vi "variantCtrlIoType.vi"(4 "isRequired (T)":bool=TRUE, 6 "menu in (get)":enum16{"get", "set"}(ring), 8 "error in":errorcluster, 9 "IoType in":T1=enum."DI", 11 "variant in":variant) -> (0 "error out":errorcluster, 1 "IoType out":T1=enum."DI", 2 "found/replaced":bool, 3 "variant out":variant)   [LabVIEW 2024]
uses:
  controls/enum.io.type.ctl
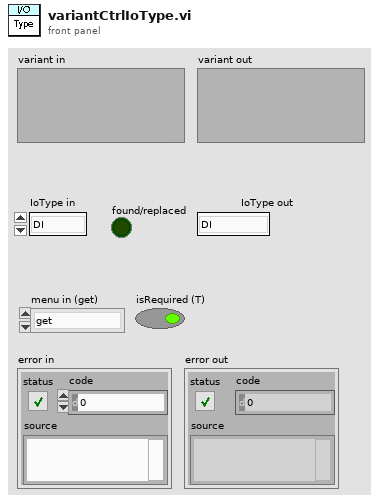
[diagram p1: front panel]
types:
  T1 = typedef "enum.io.type.ctl" = enum16{"Type", "DI", "DO", "AI", "AO", "VL", "BUF"}
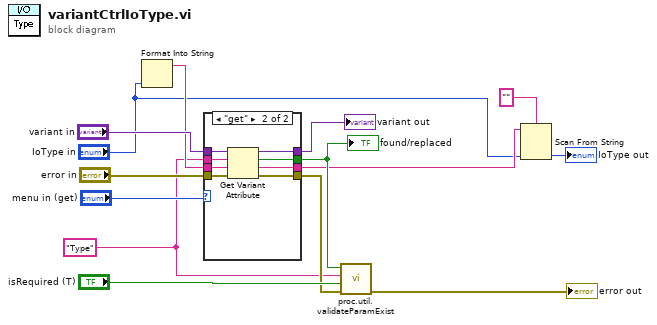
[diagram p0: block diagram]
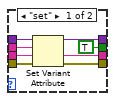
[diagram p2: hidden frame]
diagram:
  w1 = "Type"
  n1 = Format Into String("IoType in") -> (resulting string=w6:string)  [unwired: 3 in, 1 out]
  n2 = case shown="\"get\"" "menu in (get)" {
    tunnel: "error in" -> [w21 w29]
    tunnel: w6 -> [w16 w28]
    tunnel: "variant in" -> [w20 w27]
    tunnel: [w19 w26] -> w8
    tunnel: [TRUE w25] -> w9
    tunnel: [w18 w24] -> w12
    tunnel: w1 -> [w17 w23]
    tunnel: [w16 w22] -> w5
    frame "set" {
      n3 = Set Variant Attribute(Variant=w20, name=w17, value=w16, error in=w21) -> (Variant out=w18:variant, error out=w19:errorcluster)  [unwired: 1 out]
    }
    frame "get" {
      n4 = Get Variant Attribute(Variant=w27, name=w23, default value (empty Variant)=w28, error in=w29) -> (duplicate Variant=w24:variant, found=w25:bool, value=w22:string, error out=w26:errorcluster)
    }
  }
  "found/replaced" <- w9
  "variant out" <- w12
  n5 = call "proc.util.validateParamExist.vi"("error in"=w8, "isRequired"="isRequired (T)", "Param Label"=w1, "isFound"=w9) -> ("error out"=→"error out":errorcluster)  [unwired: 7 in]
  n6 = Scan From String(format string="", input string=w5, default 1="IoType in") -> (output 1=→"IoType out":T1)  [unwired: 2 in, 3 out]
